vi "LED blinking VI.vi"(6 "Wait time(ms)":dbl, 7 "Blinking/not blinking":bool, 8 "Blue":dbl, 9 "Green":dbl, 10 "Red":dbl, 11 "CANifierDevRef":T1) -> ()   [LabVIEW 2019]
uses:
  <vilib>/Rock Robotics/WPI/ThirdParty/Phoenix-LabVIEW/CANifier/CTRE_CANifier_DeviceRef.ctl
  <vilib>/Rock Robotics/WPI/ThirdParty/Phoenix-LabVIEW/CANifier/CTRE_CANifier_LEDChannel.ctl
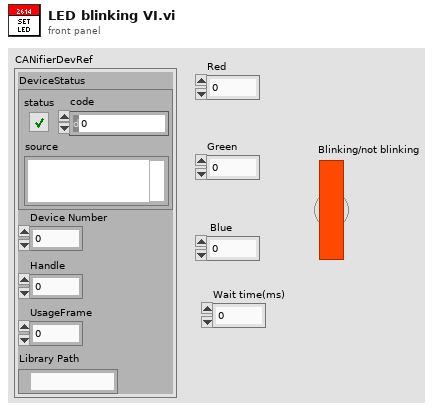
[diagram p1: front panel]
types:
  T1 = typedef "CTRE_CANifier_DeviceRef.ctl" = cluster{"DeviceStatus":errorcluster, "Device Number":u8, "Handle":u64, "UsageFrame":u32, "Library Path":path}
  T2 = typedef "CTRE_CANifier_LEDChannel.ctl" = enum32{"LEDChannelA", "LEDChannelB", "LEDChannelC"}
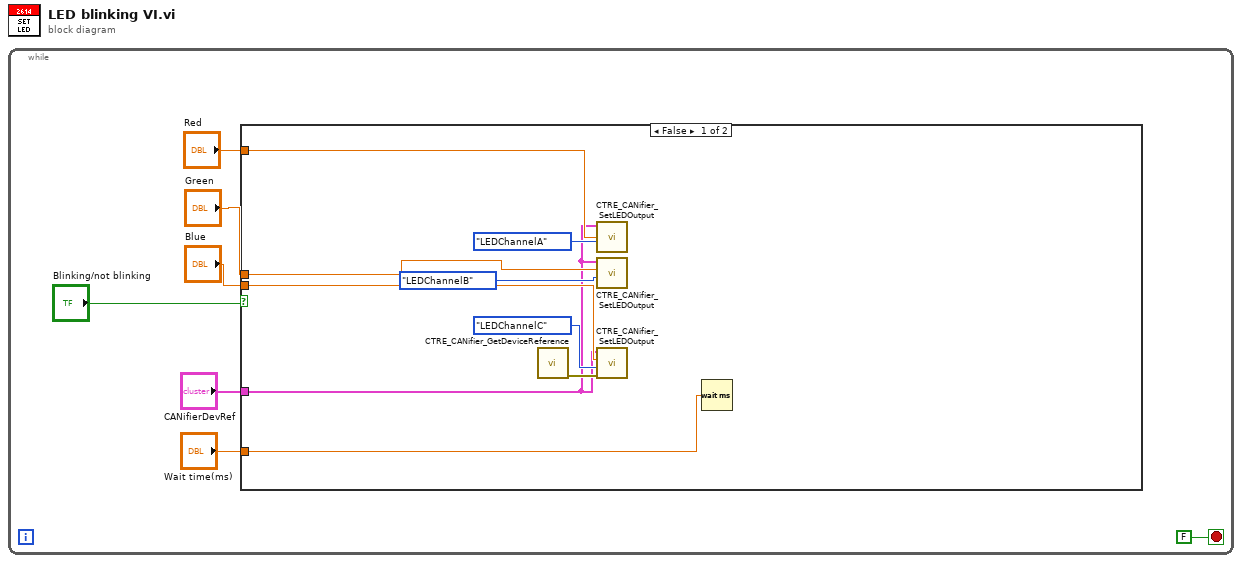
[diagram p0: block diagram]
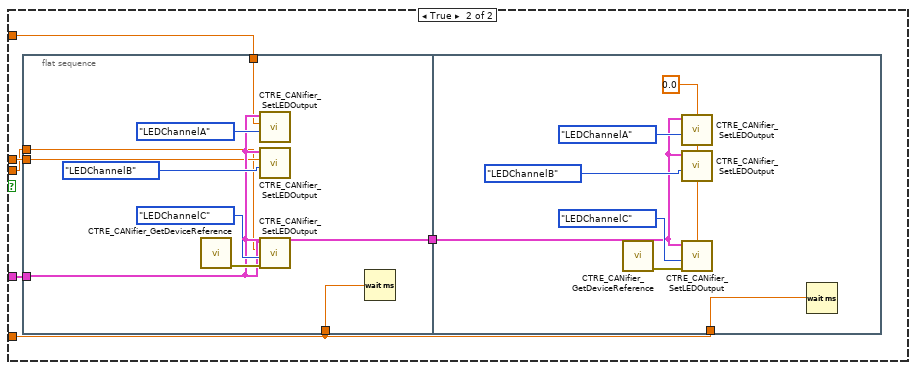
[diagram p2: hidden frame]
diagram:
  n1 = while {
    stop <- FALSE stop-if-true
    n2 = case shown="False" "Blinking/not blinking" {
      tunnel: "CANifierDevRef" -> [w8 w21]
      tunnel: "Red" -> [w12 w20]
      tunnel: "Green" -> [w10 w19]
      tunnel: "Blue" -> [w11 w18]
      tunnel: "Wait time(ms)" -> [w9 w17]
      frame False {
        n3 = call <vilib>:"CTRE_CANifier_GetDeviceReference.vi"() -> ("error out"=w16:errorcluster)  [unwired: 10 in, 1 out]
        n4 = call <vilib>:"CTRE_CANifier_SetLEDOutput.vi"("LEDChannel"=CTRE_CANifier_LEDChannel."LEDChannelA", "Percent Output"=w12, "CANifierDevRef"=w8) -> ()  [unwired: 7 in, 2 out]
        n5 = call <vilib>:"CTRE_CANifier_SetLEDOutput.vi"("LEDChannel"=CTRE_CANifier_LEDChannel."LEDChannelB", "Percent Output"=w10, "CANifierDevRef"=w8) -> ()  [unwired: 7 in, 2 out]
        n6 = call <vilib>:"CTRE_CANifier_SetLEDOutput.vi"("error in"=w16, "LEDChannel"=CTRE_CANifier_LEDChannel."LEDChannelC", "Percent Output"=w11, "CANifierDevRef"=w8) -> ()  [unwired: 6 in, 2 out]
        n7 = Wait (ms)(milliseconds to wait=w9) -> ()  [unwired: 1 out]
      }
      frame True {
        n8 = flat-sequence {
          tunnel: w21 -> [w27]
          tunnel: [w27] -> w22
          tunnel: w20 -> [w26]
          tunnel: w19 -> [w25]
          tunnel: w18 -> [w24]
          tunnel: w17 -> [w23]
          tunnel: w22 -> [w34]
          tunnel: w17 -> [w32]
          frame #0 {
            n9 = call <vilib>:"CTRE_CANifier_GetDeviceReference.vi"() -> ("error out"=w31:errorcluster)  [unwired: 10 in, 1 out]
            n10 = call <vilib>:"CTRE_CANifier_SetLEDOutput.vi"("LEDChannel"=CTRE_CANifier_LEDChannel."LEDChannelA", "Percent Output"=w26, "CANifierDevRef"=w27) -> ()  [unwired: 7 in, 2 out]
            n11 = call <vilib>:"CTRE_CANifier_SetLEDOutput.vi"("LEDChannel"=CTRE_CANifier_LEDChannel."LEDChannelB", "Percent Output"=w25, "CANifierDevRef"=w27) -> ()  [unwired: 7 in, 2 out]
            n12 = call <vilib>:"CTRE_CANifier_SetLEDOutput.vi"("error in"=w31, "LEDChannel"=CTRE_CANifier_LEDChannel."LEDChannelC", "Percent Output"=w24, "CANifierDevRef"=w27) -> ()  [unwired: 6 in, 2 out]
            n13 = Wait (ms)(milliseconds to wait=w23) -> ()  [unwired: 1 out]
          }
          frame #1 {
            w33 = 0.0
            n14 = call <vilib>:"CTRE_CANifier_GetDeviceReference.vi"() -> ("error out"=w38:errorcluster)  [unwired: 10 in, 1 out]
            n15 = call <vilib>:"CTRE_CANifier_SetLEDOutput.vi"("LEDChannel"=CTRE_CANifier_LEDChannel."LEDChannelA", "Percent Output"=w33, "CANifierDevRef"=w34) -> ()  [unwired: 7 in, 2 out]
            n16 = call <vilib>:"CTRE_CANifier_SetLEDOutput.vi"("LEDChannel"=CTRE_CANifier_LEDChannel."LEDChannelB", "Percent Output"=w33, "CANifierDevRef"=w34) -> ()  [unwired: 7 in, 2 out]
            n17 = call <vilib>:"CTRE_CANifier_SetLEDOutput.vi"("error in"=w38, "LEDChannel"=CTRE_CANifier_LEDChannel."LEDChannelC", "Percent Output"=w33, "CANifierDevRef"=w34) -> ()  [unwired: 6 in, 2 out]
            n18 = Wait (ms)(milliseconds to wait=w32) -> ()  [unwired: 1 out]
          }
        }
      }
    }
  }
